vi "Query-Acquisition-type.vi"(8 "error in":errorcluster, 11 "Data ref. in":refnum<data-value>) -> (0 "error IO":errorcluster, 2 "Hardware acquisiton?":bool, 3 "Data ref.":refnum<data-value>)   [LabVIEW 2013, in "CameraVision.lvlib" / "CV-Main.lvclass"]
uses:
  CV-Main.lvclass
  CV-Main.lvclass/CV-Main.ctl
  Acquisition/CV-Acquisition.lvclass/CV-Acquisition.ctl
  Read Acquis params.vi
  Acquisition/Read Image paths.vi
  Acquisition/CV-Acquisition.lvclass
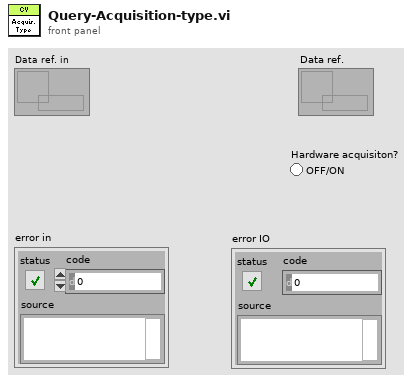
[diagram p1: front panel]
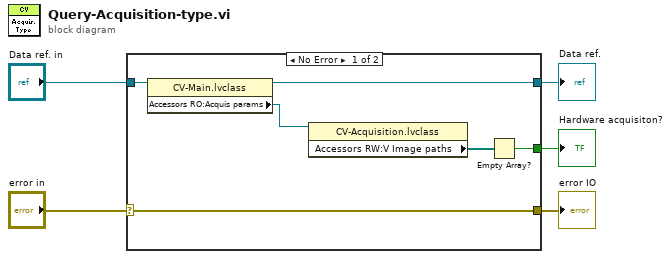
[diagram p0: block diagram]
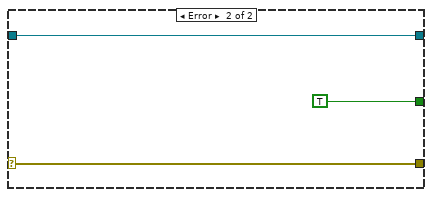
[diagram p2: hidden frame]
diagram:
  n1 = case shown="No Error" "error in" {
    selector: "error in" -> [w10 w14]
    tunnel: "Data ref. in" -> [w7 w13]
    tunnel: [w10 w14] -> w3
    tunnel: [w6 w13] -> w2
    tunnel: [w8 TRUE ("empty?")] -> w1
    frame No Error {
      n2 = property class="CV-Main.lvclass"(reference=w7) -> (reference out=w6:refnum<data-value>, "Accessors RO:Acquis params"=w11:refnum<data-value>)  [unwired: 1 in, 1 out]
      n3 = property class="CV-Acquisition.lvclass"(reference=w11) -> ("Accessors RW:V Image paths"=w9:path[])  [unwired: 1 in, 2 out]
      n4 = Empty Array?(array=w9) -> (empty?=w8:bool)
    }
    frame Error {
    }
  }
  "error IO" <- w3
  "Data ref." <- w2
  "Hardware acquisiton?" <- w1
